vi "Write offset.vi"(8 "error in (no error)":errorcluster, 10 "Offset":i16, 11 "FPGA Refs in":T1) -> (0 "error out":errorcluster, 3 "FPGA Refs out":T1)   [LabVIEW 2017, in "Piezo Controller.lvlib"]
uses:
  Piezo Controller.lvlib
  FPGA Refs.ctl
  <instrlib>/_niInstr/FIFO Register Bus/v1/Host/niInstr FIFO Register Bus v1 Host.lvclass
  C:/Program Files (x86)/National Instruments/LabVIEW 2017/instr.lib/_niInstr/Instruction Framework/v1/Host/Instruction Target/niInstr Instruction Target v1 Host.lvclass
  <instrlib>/_niInstr/Instruction Framework/v1/Host/Instruction Framework Context/niInstr Instruction Framework Context v1 Host.lvclass
  <instrlib>/_niInstr/Instruction Framework/v1/Host/Instruction Target/niInstr Instruction Target v1 Host.lvclass
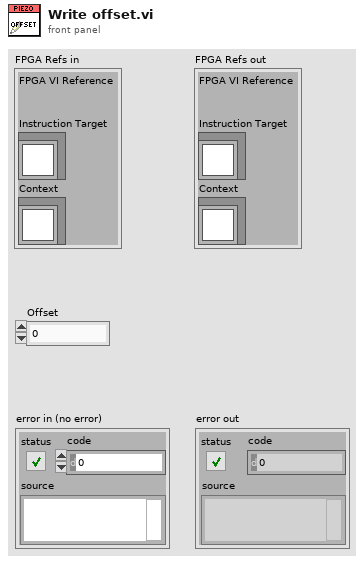
[diagram p1: front panel]
types:
  T1 = typedef "Piezo Controller.lvlib/FPGA Refs.ctl" = cluster{"FPGA VI Reference":refnum<k20>, "Instruction Target":refnum<class "niInstr FIFO Register Bus v1 Host.lvclass">, "Context":refnum<class "niInstr Instruction Framework Context v1 Host.lvclass">}
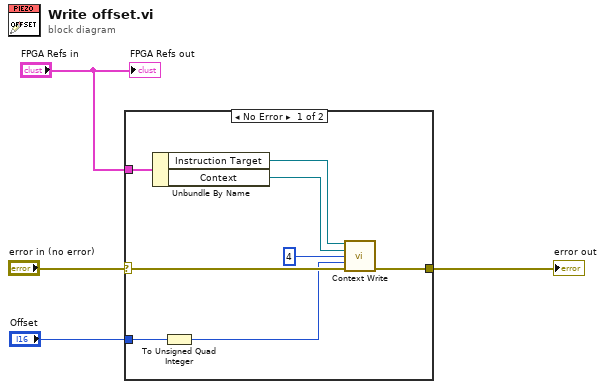
[diagram p0: block diagram]
diagram:
  n1 = case shown="No Error" "error in (no error)" {
    selector: "error in (no error)" -> [w12 w13]
    tunnel: [w11 w13] -> w3
    tunnel: "FPGA Refs in" -> [w10 _]
    tunnel: "Offset" -> [w6 _]
    frame No Error {
      n2 = Unbundle By Name(w10) -> ("Instruction Target"=w8:refnum<class "niInstr FIFO Register Bus v1 Host.lvclass">, "Context"=w9:refnum<class "niInstr Instruction Framework Context v1 Host.lvclass">)
      n3 = To Unsigned Quad Integer(1:w6) -> (0:w5:u64)
      n4 = call <instrlib>:"Context Write.vi"("instruction target in"=w8, "context in"=w9, "address"=u64 4, "data"=w5, "error in"=w12) -> ("error out"=w11:errorcluster)  [unwired: 8 in, 2 out]
    }
    frame Error {
    }
  }
  "error out" <- w3
  "FPGA Refs out" <- "FPGA Refs in"
